vi "Start.vi"(8 "error in (no error)":errorcluster, 11 "VeriStand Data Sharing Framework in":refnum<class "VeriStand DSF.lvclass">=refnum) -> (0 "error out":errorcluster, 3 "VeriStand Data Sharing Framework out":refnum<class "VeriStand DSF.lvclass">)   [LabVIEW 2019, in "DSF Engine.lvlib" / "VeriStand DSF.lvclass"]
uses:
  VeriStand DSF.lvclass
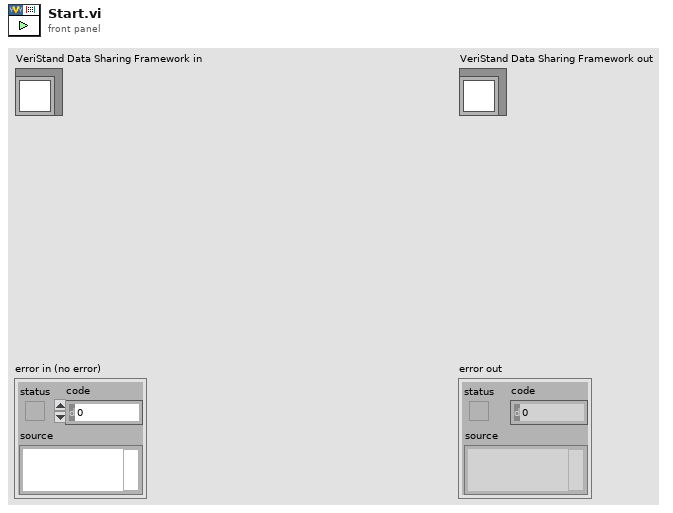
[diagram p1: front panel]
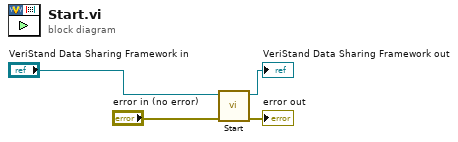
[diagram p0: block diagram]
diagram:
  n1 = call-parent "Start.vi"("error in (no error)"="error in (no error)", "Framework in"="VeriStand Data Sharing Framework in") -> ("error out"=→"error out":errorcluster, "Framework out"=→"VeriStand Data Sharing Framework out":refnum<class "VeriStand DSF.lvclass">)  [unwired: 8 in]
